vi "Autunomous Initilization.vi"() -> (0 "errror out":errorcluster)   [LabVIEW 2019]
uses:
  Utility VIs/Refnum Names.vi
  <vilib>/Rock Robotics/WPI/Utilities/WPI_GetSetVariantRefNum.vi
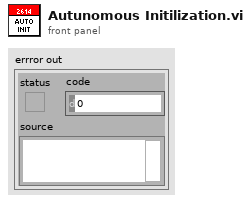
[diagram p1: front panel]
types:
  T1 = typedef "CTRE_PigeonIMU_DeviceRef.ctl" = cluster{"DeviceStatus":errorcluster, "Device Number":u8, "Type":T2, "Device ID":u32, "Handle":u64, "UsageFrame":u32, "Library Path":path}
  T2 = typedef "CTRE_PigeonIMU_ConnectionType.ctl" = u32
  T3 = typedef "WPI_CompressorDevRef.ctl" = cluster{"DevStatus":errorcluster, "Pneumatics Control Module":u8}
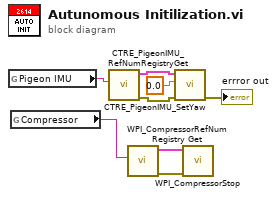
[diagram p0: block diagram]
diagram:
  n1 = global read "Refnum Names.vi" "Pigeon IMU"() -> (w8:string)
  n2 = global read "Refnum Names.vi" "Compressor"() -> (w3:string)
  n3 = call <vilib>:"CTRE_PigeonIMU_RefNumRegistryGet.vi"("refnum name"=w8) -> ("error out"=w5:errorcluster, "PigeonIMUDevRef"=w6:T1)  [unwired: 9 in]
  n4 = call <vilib>:"WPI_CompressorRefNum Registry Get.vi"("refnum name"=w3) -> ("error out"=w1:errorcluster, "CompressorDevRef"=w2:T3)  [unwired: 9 in]
  n5 = call <vilib>:"CTRE_PigeonIMU_SetYaw.vi"("error in (no error)"=w5, "Value"=0.0, "PigeonIMUDevRef"=w6) -> ("error out"=→"errror out":errorcluster)  [unwired: 7 in, 1 out]
  n6 = call <vilib>:"WPI_CompressorStop.vi"("error in (no error)"=w1, "CompressorDevRef"=w2) -> ()  [unwired: 8 in, 2 out]
